vi "Autonomous Independent.vi"() -> ()   [LabVIEW 2017]
doc: "This VI is called when autonomous begins, and will automatically be terminated when autonomous ends. You can carry out timed or sensor driven robot movement independently without needing to return to the caller."
uses:
  <vilib>/Rock Robotics/WPI/RobotDrive/WPI_RobotDriveArcadeDrive_Standard(NoSaturation).vi
  <vilib>/Rock Robotics/Network Tables/NT Write Numeric Array.vi
  <vilib>/Rock Robotics/Network Tables/NT Read String.vi
panel:
  out "Current Movement, for debugging":T1 {"Y Joystick Value" scale=1.0..-1.0; "X Joystick Value" scale=-1.0..1.0}
  in  "Array of robot movements":T2(array[cluster])=[{"X Joystick Value"=0.39393939393939403, "Y Joystick Value"=0.0, "Delay (sec)"=1.0, "Movement Name"="turn"}, {"X Joystick Value"=-0.3737373737373737, "Y Joystick Value"=0.0, "Delay (sec)"=1.0, "Movement Name"="turn back"}] {"Y Joystick Value" scale=1.0..-1.0; "X Joystick Value" scale=-1.0..1.0}
  # "Be sure to right-click and choose Data Operations>>Make Current Value default if you want to save the array values with the VI"
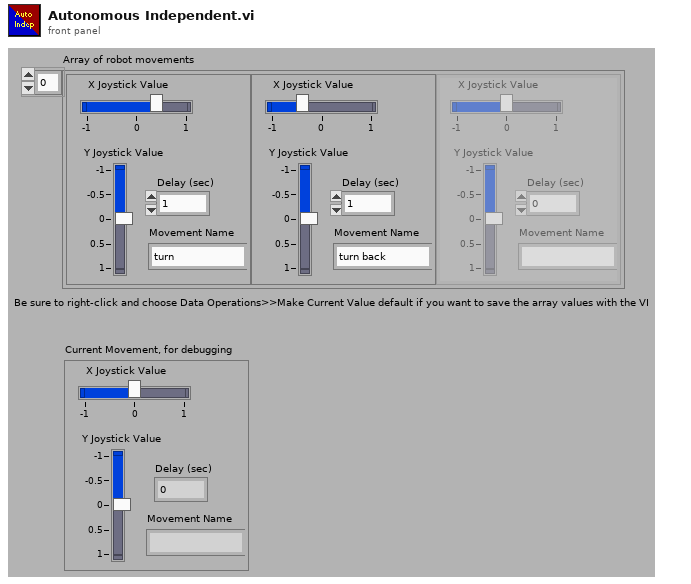
[diagram p1: front panel]
types:
  T1 = cluster{"X Joystick Value":dbl, "Y Joystick Value":dbl, "Delay (sec)":dbl, "Movement Name":string}
  T2 = cluster{"X Joystick Value":dbl, "Y Joystick Value":dbl, "Delay (sec)":dbl, "Movement Name":string}[]
  T3 = typedef "WPI_JoystickDevRef.ctl" = cluster{"Device":T4}
  T4 = typedef "WPI_JoystickDeviceEnum.ctl" = enum16{"USB 0", "USB 1", "USB 2", "USB 3", "USB 4", "USB 5"}
  T5 = typedef "WPI_RobotDriveDevRef.ctl" = cluster{"DevStatus":errorcluster, "Motors[]":T6[], "Square Inputs":bool, "Max Output":dbl}
  T6 = typedef "WPI_MotorControlDeviceRef.ctl" = cluster{"DeviceStatus":errorcluster, "Type":T7, "PWM":cluster{"PWM Channel":T8, "DeadBand":T9}, "CAN":cluster{"Device Number":u8, "SetOutput VI Ref":variant, "GetOutput VI Ref":variant, "Enable VI Ref":variant, "Disable VI Ref":variant, "Data":variant}, "Invert":bool, "DIO PWM":cluster{"PWM \"Enable\" Channel":T8, "DIOChannel":T10, "PWM Rate":dbl}}
  T7 = typedef "WPI_MotorControlType.ctl" = enum16{"PWM", "CAN", "DIO PWM"}
  T8 = typedef "FPGA_DIOPWMChannel.ctl" = enum8{"PWM 0", "PWM 1", "PWM 2", "PWM 3", "PWM 4", "PWM 5", "PWM 6", "PWM 7", "PWM 8", "PWM 9", "PWM MXP 0", "PWM MXP 1", "PWM MXP 2", "PWM MXP 3", "PWM MXP 4", "PWM MXP 5", "PWM MXP 6", "PWM MXP 7", "PWM MXP 8", "PWM MXP 9", "Invalid"}
  T9 = typedef "WPI_PWMDeadband.ctl" = cluster{"Name":string, "maxPositivePwm":i32, "minPositivePwm":i32, "centerPwm":i32, "maxNegativePwm":i32, "minNegativePwm":i32, "angularRange":u16}
  T10 = typedef "FPGA_DIOChannel.ctl" = enum8{"DIO 0", "DIO 1", "DIO 2", "DIO 3", "DIO 4", "DIO 5", "DIO 6", "DIO 7", "DIO 8", "DIO 9", "DIO MXP 0", "DIO MXP 1", "DIO MXP 2", "DIO MXP 3", "DIO MXP 4", "DIO MXP 5", "DIO MXP 6", "DIO MXP 7", "DIO MXP 8", "DIO MXP 9", "DIO MXP 10", "DIO MXP 11", "DIO MXP 12", "DIO MXP 13", "DIO MXP 14", "DIO MXP 15", "SPI Port CS1", "SPI Port CS2", "SPI Port CS3", "SPI Port MISO", "SPI Port MOSI", "Invalid"}
  T11 = typedef "WPI_GyroDevRef.ctl" = cluster{"DevStatus":errorcluster, "Analog Channel":T12, "Gain (VoltsPerDegree/Second)":dbl, "Gyro Type":enum16{"Analog", "XRS450"}, "Handle":i32, "SPI Bus":T13, "Device Found":bool, "Sample Rate":dbl, "Calibrate On Open":bool, "Offset":dbl}
  T12 = typedef "FPGA_AIChannel.ctl" = enum8{"AI 0", "AI 1", "AI 2", "AI 3", "AI MXP 0", "AI MXP 1", "AI MXP 2", "AI MXP 3", "Invalid"}
  T13 = typedef "spi_bus.ctl" = enum16{"SPI On-Board, CS0", "SPI On-Board, CS1", "SPI On-Board, CS2", "SPI On-Board, CS3", "SPI MXP", "Invalid"}
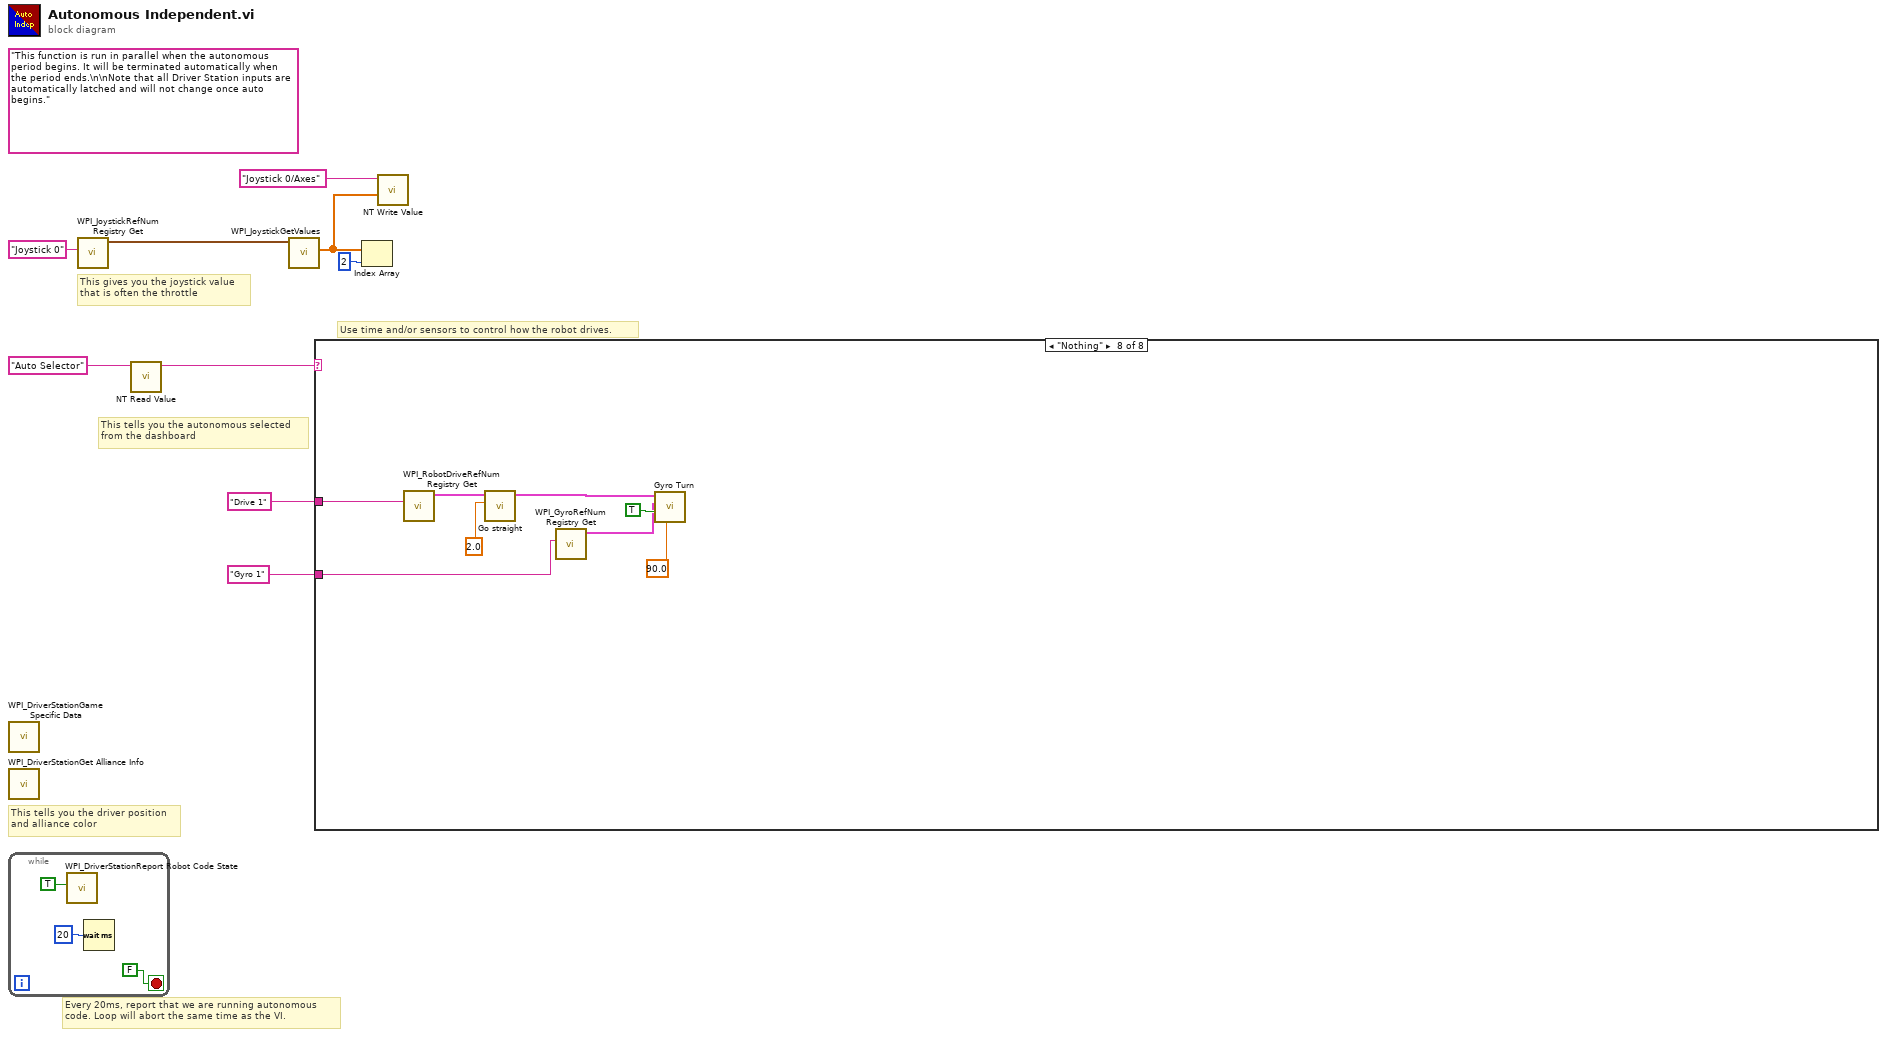
[diagram p0: block diagram]
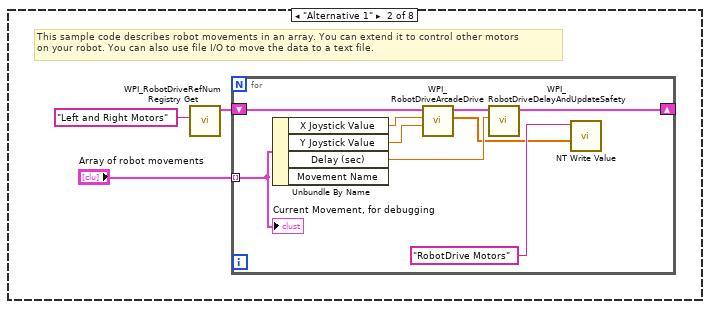
[diagram p3: hidden frame]
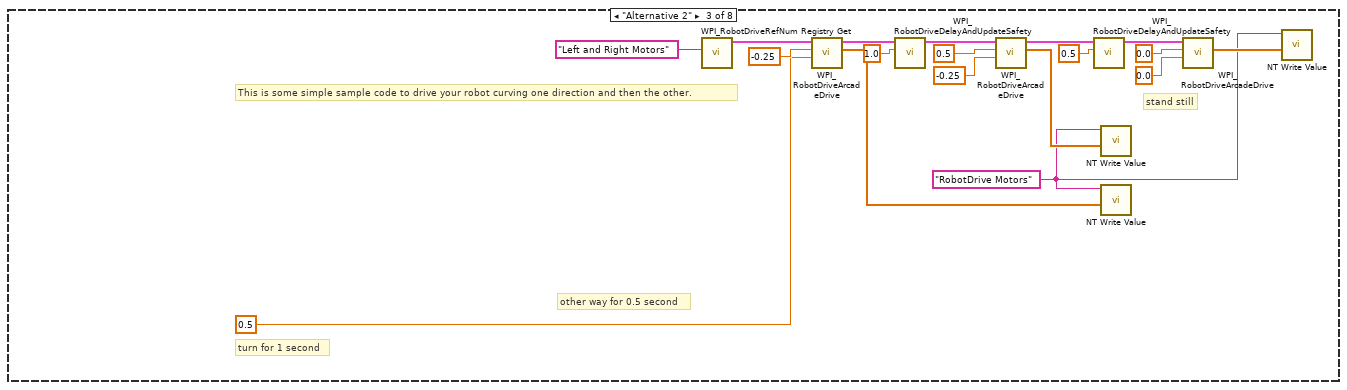
[diagram p4: hidden frame]
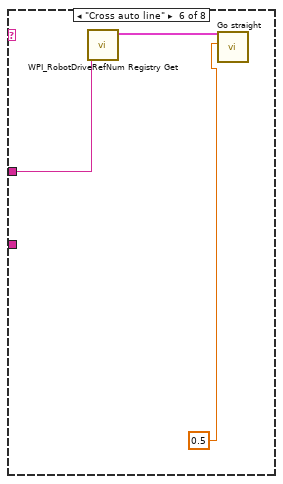
[diagram p7: hidden frame]
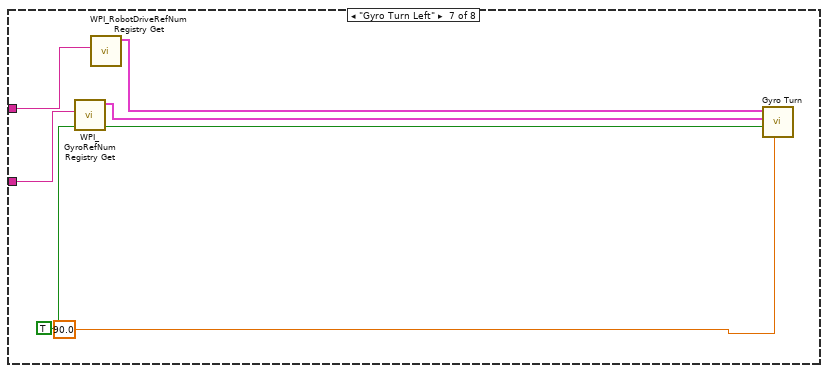
[diagram p8: hidden frame]
diagram:
  (unwired) "This function is run in parallel when the autonomous period begins. It will be terminated automatically when the period ends.\n\nNote that all Driver Station inputs are automatically latched and will not change once auto begins."
  # "This tells you the autonomous selected\nfrom the dashboard"
  # "Every 20ms, report that we are running autonomous\ncode. Loop will abort the same time as the VI."
  # "This gives you the joystick value\nthat is often the throttle"
  # "Use time and/or sensors to control how the robot drives."
  # "This tells you the driver position\nand alliance color"
  n1 = call <vilib>:"WPI_DriverStationGame Specific Data.vi"() -> ()  [unwired: 11 in, 1 out]
  n2 = call <vilib>:"WPI_DriverStationGet Alliance Info.vi"() -> ()  [unwired: 12 out]
  n3 = while {
    stop <- FALSE stop-if-true
    n4 = call <vilib>:"WPI_DriverStationReport Robot Code State.vi"("Autonomous"=TRUE) -> ()  [unwired: 10 in, 1 out]
    n5 = Wait (ms)(milliseconds to wait=u32 20) -> ()  [unwired: 1 out]
  }
  n6 = call <vilib>:"WPI_JoystickRefNum Registry Get.vi"("refnum name"="Joystick 0") -> ("JoystickDevRef"=w8:T3)  [unwired: 1 in, 9 out]
  n7 = call-poly <vilib>:"NT Read Value.vi"("Name"="Auto Selector") -> ("String"=w3:string)  [unwired: 9 in, 1 out]
  n8 = call <vilib>:"WPI_JoystickGetValues.vi"("JoystickDevRef"=w8) -> ("Axes"=w5:dbl[])  [unwired: 6 in, 4 out]
  n9 = case shown="\"Nothing\"" w3 {
    tunnel: "Drive 1" ("refnum name") -> [_ _ _ _ _ w43 w46 w58]
    tunnel: "Gyro 1" ("refnum name") -> [_ _ _ _ _ _ w47 w52]
    frame Default {
      # "You can put your main auto here, or you can right-click on the case and make any\nother frame be the default case."
      # "This is the frame that will execute if no selection is made, or if it is not recognized"
    }
    frame "Alternative 1" {
      # "This sample code describes robot movements in an array. You can extend it to control other motors\non your robot. You can also use file I/O to move the data to a text file."
      n10 = call <vilib>:"WPI_RobotDriveRefNum Registry Get.vi"("refnum name"="Left and Right Motors") -> ("RobotDriveDevRef"=w14:T5)  [unwired: 1 in, 9 out]
      n11 = for {
        shift-right: [w22] -> _
        shift-left: w14 -> [w23]
        tunnel: "Array of robot movements" -> [w18] mode=indexing
        n12 = Unbundle By Name(w18) -> ("X Joystick Value"=w21:dbl, "Y Joystick Value"=w20:dbl, "Delay (sec)"=w19:dbl)  [unwired: 1 out]
        n13 = call-poly <vilib>:"WPI_RobotDriveArcadeDrive.vi"("Y axis value"=w20, "X axis value"=w21, "RobotDriveDevRef"=w23) -> ("Motor Values"=w16:dbl[], "RobotDriveDevRef"=w24:T5)  [unwired: 1 in, 6 out]
        n14 = call <vilib>:"WPI_RobotDriveDelayAndUpdateSafety.vi"("Delay (s)"=w19, "RobotDriveDevRef"=w24) -> ("RobotDriveDevRef 2"=w22:T5)  [unwired: 8 in, 1 out]
        n15 = call-poly <vilib>:"NT Write Value.vi"("Numeric Array"=w16, "Name"="RobotDrive Motors") -> ()  [unwired: 9 in, 1 out]
        "Current Movement, for debugging" <- w18
      }
    }
    frame "Alternative 2" {
      w26 = "RobotDrive Motors" ("Name")
      # "This is some simple sample code to drive your robot curving one direction and then the other."
      # "stand still"
      # "other way for 0.5 second"
      # "turn for 1 second"
      n16 = call <vilib>:"WPI_RobotDriveRefNum Registry Get.vi"("refnum name"="Left and Right Motors") -> ("RobotDriveDevRef"=w42:T5)  [unwired: 1 in, 9 out]
      n17 = call-poly <vilib>:"WPI_RobotDriveArcadeDrive.vi"("Y axis value"=0.5 ("X axis value"), "X axis value"=-0.25, "RobotDriveDevRef"=w42) -> ("Motor Values"=w25:dbl[], "RobotDriveDevRef"=w35:T5)  [unwired: 1 in, 6 out]
      n18 = call <vilib>:"WPI_RobotDriveDelayAndUpdateSafety.vi"("Delay (s)"=1.0, "RobotDriveDevRef"=w35) -> ("RobotDriveDevRef 2"=w36:T5)  [unwired: 8 in, 1 out]
      n19 = call-poly <vilib>:"WPI_RobotDriveArcadeDrive.vi"("Y axis value"=-0.25 ("X axis value"), "X axis value"=0.5, "RobotDriveDevRef"=w36) -> ("Motor Values"=w27:dbl[], "RobotDriveDevRef"=w37:T5)  [unwired: 1 in, 6 out]
      n20 = call <vilib>:"WPI_RobotDriveDelayAndUpdateSafety.vi"("Delay (s)"=0.5, "RobotDriveDevRef"=w37) -> ("RobotDriveDevRef 2"=w38:T5)  [unwired: 8 in, 1 out]
      n21 = call-poly <vilib>:"NT Write Value.vi"("Numeric Array"=w27, "Name"=w26) -> ()  [unwired: 9 in, 1 out]
      n22 = call-poly <vilib>:"NT Write Value.vi"("Numeric Array"=w25, "Name"=w26) -> ()  [unwired: 9 in, 1 out]
      n23 = call-poly <vilib>:"WPI_RobotDriveArcadeDrive.vi"("Y axis value"=0.0 ("X axis value"), "X axis value"=0.0, "RobotDriveDevRef"=w38) -> ("Motor Values"=w28:dbl[])  [unwired: 1 in, 7 out]
      n24 = call-poly <vilib>:"NT Write Value.vi"("Numeric Array"=w28, "Name"=w26) -> ()  [unwired: 9 in, 1 out]
    }
    frame "Your Turn" {
    }
    frame "Do Nothing" {
    }
    frame "Cross auto line" {
      n25 = call <vilib>:"WPI_RobotDriveRefNum Registry Get.vi"("refnum name"=w43) -> ("RobotDriveDevRef"=w44:T5)  [unwired: 9 in, 1 out]
      n26 = call "Go straight.vi"("Delay (s)"=0.5, "RobotDriveDevRef in"=w44) -> ()  [unwired: 9 in, 1 out]
    }
    frame "Gyro Turn Left" {
      n27 = call <vilib>:"WPI_GyroRefNum Registry Get.vi"("refnum name"=w47) -> ("GyroDevRef"=w50:T11)  [unwired: 9 in, 1 out]
      n28 = call <vilib>:"WPI_RobotDriveRefNum Registry Get.vi"("refnum name"=w46) -> ("RobotDriveDevRef"=w51:T5)  [unwired: 9 in, 1 out]
      n29 = call "Gyro Turn.vi"("degrees"=90.0 ("y"), "If right"=TRUE, "GyroDevRef"=w50, "RobotDriveDevRef in"=w51) -> ()  [unwired: 7 in, 1 out]
    }
    frame "Nothing" {
      n30 = call <vilib>:"WPI_RobotDriveRefNum Registry Get.vi"("refnum name"=w58) -> ("RobotDriveDevRef"=w57:T5)  [unwired: 9 in, 1 out]
      n31 = call "Go straight.vi"("Delay (s)"=2.0, "RobotDriveDevRef in"=w57) -> ("RobotDriveDevRef out"=w56:T5)  [unwired: 9 in]
      n32 = call <vilib>:"WPI_GyroRefNum Registry Get.vi"("refnum name"=w52) -> ("GyroDevRef"=w53:T11)  [unwired: 9 in, 1 out]
      n33 = call "Gyro Turn.vi"("degrees"=90.0, "If right"=TRUE, "GyroDevRef"=w53, "RobotDriveDevRef in"=w56) -> ()  [unwired: 7 in, 1 out]
    }
  }
  n34 = Index Array(array=w5, index=2) -> ()  [unwired: 1 out]
  n35 = call-poly <vilib>:"NT Write Value.vi"("Numeric Array"=w5, "Name"="Joystick 0/Axes") -> ()  [unwired: 9 in, 1 out]
